vi "Profile XY.vi"(8 "error in (no error)":errorcluster caption="entrée d'erreur (pas d'erreur)", 10 "Image in":T1(plugin-control), 11 "Acq Cam Basler en entrée":refnum<class "Acq Cam Basler.lvclass">) -> (0 "error out":errorcluster caption="sortie d'erreur", 2 "Image out":T1(plugin-control), 3 "Acq Cam Basler en sortie":refnum<class "Acq Cam Basler.lvclass">)   [LabVIEW 2023, in "Acq Cam Basler.lvclass"]
uses:
  Acq Cam Basler.lvclass
  Acq Cam Basler.lvclass/Acq Cam Basler.ctl
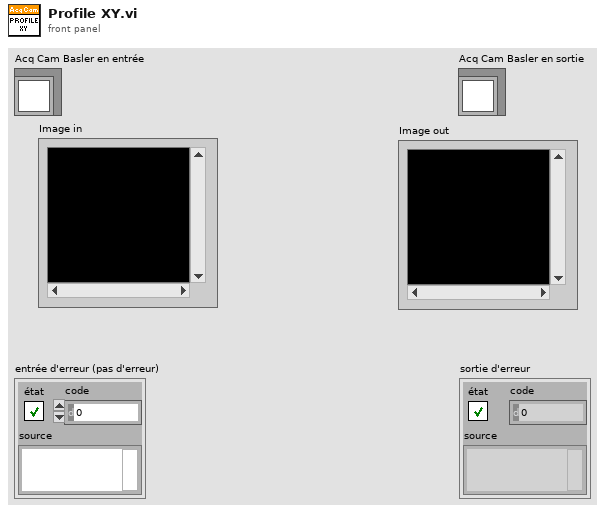
[diagram p1: front panel]
types:
  T1 = typedef "IMAQ Image.ctl" = refnum<image>
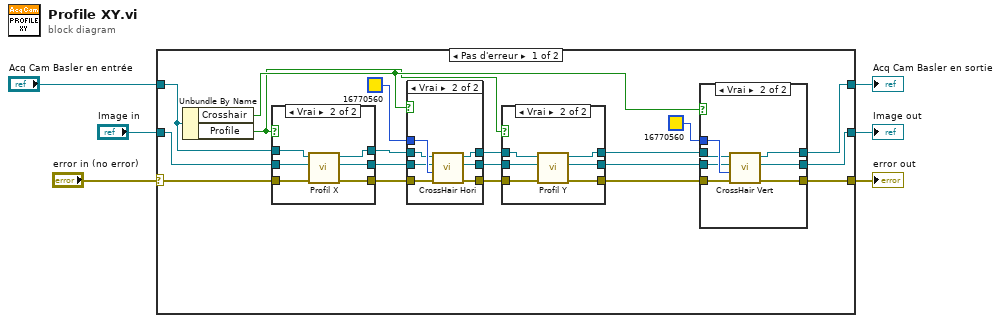
[diagram p0: block diagram]
diagram:
  n1 = case shown="Pas d'erreur" "error in (no error)" {
    selector: "error in (no error)" -> [w20 w66]
    tunnel: [w25 w66] -> w5
    tunnel: [w24 w65] -> w3
    tunnel: "Acq Cam Basler en entrée" -> [w9 w65]
    tunnel: "Image in" -> [w17 w64]
    tunnel: [w23 w64] -> w1
    frame No Error {
      n2 = Unbundle By Name(w9) -> ("Crosshair"=w8:bool, "Profile"=w7:bool)
      n3 = case shown="Vrai" w7 {
        tunnel: w20 -> [w35 w43]
        tunnel: [w35 w42] -> w19
        tunnel: [w37 w41] -> w18
        tunnel: w17 -> [w36 w40]
        tunnel: [w36 w39] -> w16
        tunnel: w9 -> [w37 w38]
        frame False {
        }
        frame True {
          n4 = call "Profil X.vi"("error in (no error)"=w43, "Image in"=w40, "Acq Cam Basler en entrée"=w38) -> ("error out"=w42:errorcluster, "Image out"=w39:T1, "Acq Cam Basler en sortie"=w41:refnum<class "Acq Cam Basler.lvclass">)  [unwired: 6 in]
        }
      }
      n5 = case shown="Vrai" w8 {
        tunnel: u32 16770560 ("Couleur Ligne Vert") -> [_ w63]
        tunnel: w19 -> [w55 w62]
        tunnel: w18 -> [w56 w61]
        tunnel: w16 -> [w54 w60]
        tunnel: [w56 w59] -> w15
        tunnel: [w54 w58] -> w13
        tunnel: [w55 w57] -> w11
        frame False {
        }
        frame True {
          n6 = call "CrossHair Hori.vi"("error in (no error)"=w62, "Couleur Ligne Hori"=w63, "Image In"=w60, "Acq Cam Basler en entrée"=w61) -> ("error out"=w57:errorcluster, "Image Out"=w58:T1, "Acq Cam Basler en sortie"=w59:refnum<class "Acq Cam Basler.lvclass">)  [unwired: 5 in]
        }
      }
      n7 = case shown="Vrai" w7 {
        tunnel: w15 -> [w28 w34]
        tunnel: [w28 w33] -> w14
        tunnel: w13 -> [w27 w32]
        tunnel: [w27 w31] -> w12
        tunnel: w11 -> [w26 w30]
        tunnel: [w26 w29] -> w10
        frame False {
        }
        frame True {
          n8 = call "Profil Y.vi"("error in (no error)"=w30, "Image in"=w32, "Acq Cam Basler en entrée"=w34) -> ("error out"=w29:errorcluster, "Image out"=w31:T1, "Acq Cam Basler en sortie"=w33:refnum<class "Acq Cam Basler.lvclass">)  [unwired: 6 in]
        }
      }
      n9 = case shown="Vrai" w8 {
        tunnel: [w46 w53] -> w25
        tunnel: [w44 w52] -> w24
        tunnel: [w45 w51] -> w23
        tunnel: u32 16770560 ("Couleur Ligne Vert") -> [_ w50]
        tunnel: w14 -> [w44 w49]
        tunnel: w12 -> [w45 w48]
        tunnel: w10 -> [w46 w47]
        frame False {
        }
        frame True {
          n10 = call "CrossHair Vert.vi"("error in (no error)"=w47, "Couleur Ligne Vert"=w50, "Image In"=w48, "Acq Cam Basler en entrée"=w49) -> ("error out"=w53:errorcluster, "Image Out"=w51:T1, "Acq Cam Basler en sortie"=w52:refnum<class "Acq Cam Basler.lvclass">)  [unwired: 5 in]
        }
      }
    }
    frame Error {
    }
  }
  "error out" <- w5
  "Acq Cam Basler en sortie" <- w3
  "Image out" <- w1
